vi "Setup.vi"(8 "error in (no error)":errorcluster, 10 "Input Method Debug":enum32{"Webcam Input", "Xbox Controller"}(tab)) -> (0 "error out":errorcluster, 2 "Input Method":enum32{"Webcam Input", "Xbox Controller"}(tab))   [LabVIEW 2016]
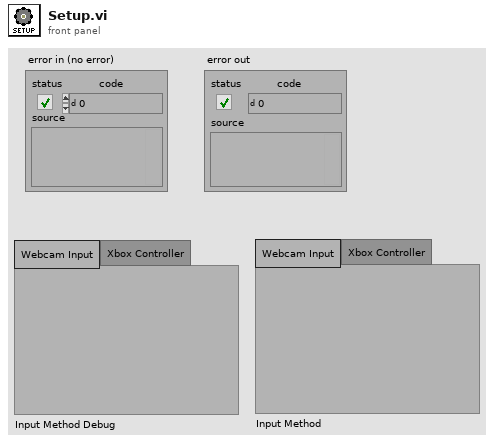
[diagram p1: front panel]
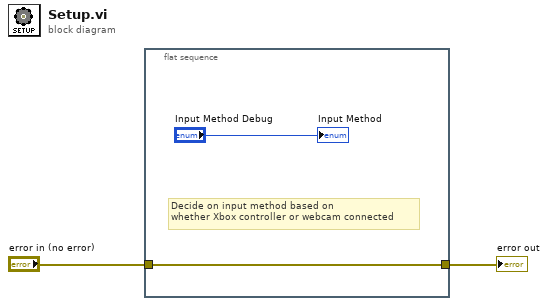
[diagram p0: block diagram]
diagram:
  n1 = flat-sequence {
    tunnel: [w4] -> w2
    tunnel: "error in (no error)" -> [w4]
    frame #0 {
      # "Decide on input method based on\nwhether Xbox controller or webcam connected"
      "Input Method" <- "Input Method Debug"
    }
  }
  "error out" <- w2
